vi "AlazarNumOfSystems.vi"(0 "error in (no error)":errorcluster) -> (1 "System Count":u32, 2 "error out":errorcluster)   [LabVIEW 2018]
doc: "Get the total number of board systems detected."
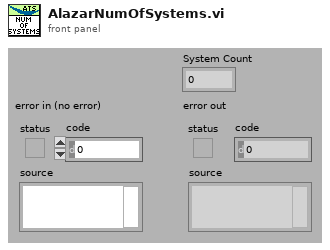
[diagram p1: front panel]
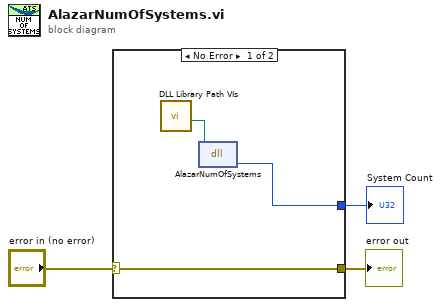
[diagram p0: block diagram]
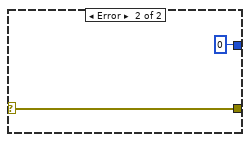
[diagram p2: hidden frame]
diagram:
  n1 = case shown="No Error" "error in (no error)" {
    selector: "error in (no error)" -> [w5 w8]
    tunnel: [w5 w8] -> w2
    tunnel: [w6 u32 0] -> w1
    frame No Error {
      n2 = call "DLL Library Path VIs.vi"() -> ("Alazar"=w4:path)  [unwired: 9 in, 2 out]
      n3 = dll-call lib="C:/Project/SerialSectOCT - FFT GPU/SerialSectOCT/Labview Software/DLL/ATSApi.dll" fn="AlazarNumOfSystems"(path in=w4) -> ("return type"=w6:u32)  [unwired: 2 in, 2 out]
    }
    frame Error {
    }
  }
  "error out" <- w2
  "System Count" <- w1
